vi "Exponential Window (DBL).vi"(2 "final value":dbl=0.1 format="%0.2f", 3 "X":dbl[](array[numeric])) -> (0 "error":i32, 1 "Windowed X":dbl[](array[numeric]))   [LabVIEW 2017, in "NI_AALPro.lvlib"]
doc: "Applies an exponential window to the input signal <B>X</B>. Wire data to the <B>X</B> input to determine the polymorphic instance to use or manually select the instance."
uses:
  NI_AALPro.lvlib
  <resource>/lvanlys.dll
panel:
  # "Exponential Window"
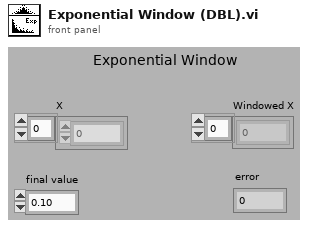
[diagram p1: front panel]
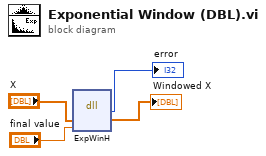
[diagram p0: block diagram]
diagram:
  n1 = dll-call lib="C:/Program Files (x86)/National Instruments/LabVIEW 2017/resource/lvanlys.*" fn="ExpWinH"("X"="X", "final"="final value") -> (→"error":i32, "X"=→"Windowed X":dbl[])  [unwired: 4 in, 2 out]
